vi "Open Build.vi"(8 "error in (no error)":errorcluster, 10 "Build specification name":string, 11 "Project Refnum":refnum<vi>) -> (0 "error out":errorcluster, 3 "DLL out":refnum<class "NI_AB_API_DLL.lvclass">)   [LabVIEW 2020, in "NI_AB_API_DLL.lvclass"]
uses:
  <vilib>/AppBuilder/AB_API/DLL/NI_AB_API_DLL.lvclass
panel:
  in  "TargetItem Refnum":refnum<vi>
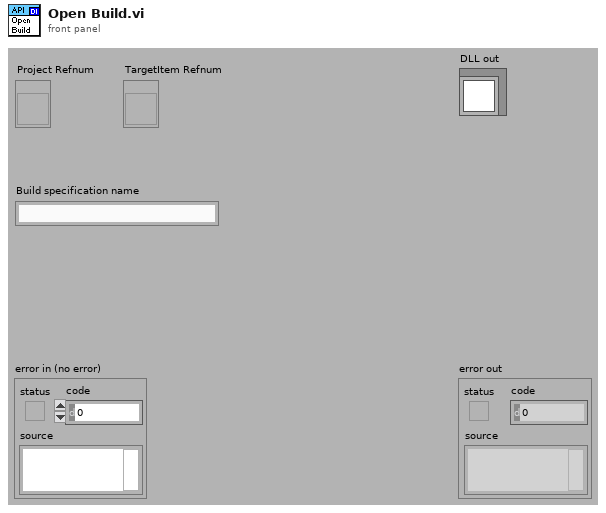
[diagram p1: front panel]
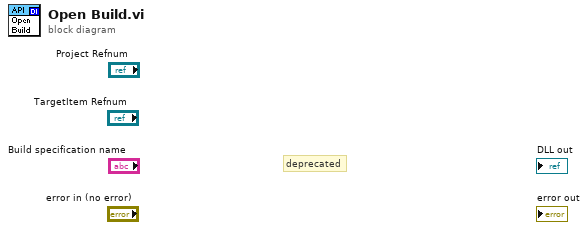
[diagram p0: block diagram]
diagram:
  # "deprecated"
